vi "2.3.vi"() -> ()   [LabVIEW 2020]
panel:
  out "Array 2":dbl[][](array[numeric])
  in  "Array":dbl[][](array[numeric])
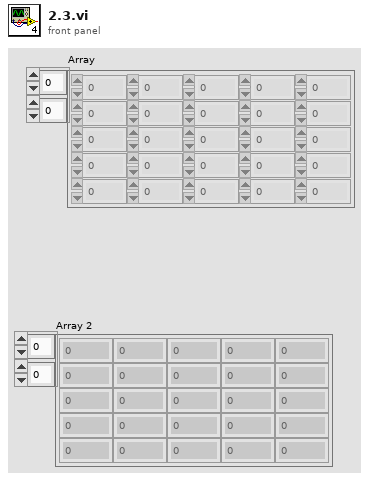
[diagram p1: front panel]
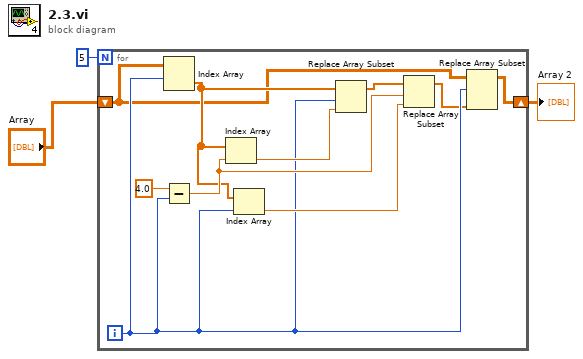
[diagram p0: block diagram]
diagram:
  n1 = for {
    N: 5 -> [_]
    shift-right: [w4] -> w1
    shift-left: "Array" -> [w5]
    i -> [w7]
    n2 = Index Array(array=w5, index (row)=w7) -> (element=w8:dbl[])  [unwired: 1 in]
    n3 = Subtract(x=4.0, y=w7) -> (x-y=w9:dbl)
    n4 = Index Array(array=w8, index=w9) -> (element=w12:dbl)
    n5 = Index Array(array=w8, index=w7) -> (element=w10:dbl)
    n6 = Replace Array Subset(array=w8, new element=w12, index=w7) -> (w11:dbl[])
    n7 = Replace Array Subset(array=w11, new element=w10, index=w9) -> (w6:dbl[])
    n8 = Replace Array Subset(array=w5, new element=w6, index (row)=w7) -> (w4:dbl[][])  [unwired: 1 in]
  }
  "Array 2" <- w1
